vi "DriveZeroRadiusTurnPlanner.vi"(4 "DrivePathPlanParams":T3={"max_velocity (in/s)"=100.0, "max_acceleration (in/s^2)"=80.0, "max_jerk (in/s^3)"=100.0, "dt(ms)"=40, "sample_count"=1000, "wheelbase_width (in)"=25.0} {"dt(ms)" items=["TrajectoryDuration_0ms"=0, "TrajectoryDuration_5ms"=5, "TrajectoryDuration_10ms"=10, "TrajectoryDuration_20ms"=20, "TrajectoryDuration_30ms"=30, "TrajectoryDuration_40ms"=40, "TrajectoryDuration_50ms"=50, "TrajectoryDuration_100ms"=100]}, 5 "Waypoints":T2[](array[typedef])) -> (1 "RightTrajectory":T1[](array[typedef]), 2 "LeftTrajectory":T1[](array[typedef]))   [LabVIEW 2018]
uses:
  PathPlannerSupport/TypeDefs/DrivePathfinderParams.ctl
  <vilib>/Rock Robotics/WPI/ThirdParty/Phoenix-LabVIEW/Motor Controller/Controls/CTRE_Phoenix_MotorControl_TrajectoryPointTimeDur.ctl
  Pathfinder/Pathfinder-LabVIEW/Pathfinder-Lib/VIs/Waypoint.ctl
  Pathfinder/Pathfinder-LabVIEW/Pathfinder-Lib/VIs/Segment.ctl
  General/MotionProfiling/TypeDefs/MotionProfileGeneratorParams.ctl
  Pathfinder/Pathfinder-LabVIEW/Pathfinder-Lib/Pathfinder.lvlib
  ArgosLib/ArgosLib.lvlib
panel:
  in  "Maximum Travel Speed (units/s)":dbl=100.0 format="%#_13g"
  in  "Velocity Ramp Time (ms)":dbl=100.0 format="%#_13g"
  in  "Acceleration Ramp Time (ms)":dbl=200.0 format="%#_13g"
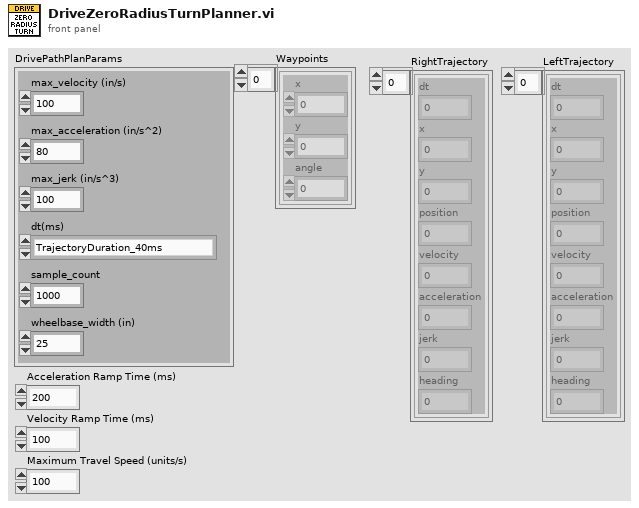
[diagram p1: front panel]
types:
  T1 = typedef "Pathfinder.lvlib/Segment.ctl" = cluster{"dt":dbl, "x":dbl, "y":dbl, "position":dbl, "velocity":dbl, "acceleration":dbl, "jerk":dbl, "heading":dbl}
  T2 = typedef "Pathfinder.lvlib/Waypoint.ctl" = cluster{"x":dbl, "y":dbl, "angle":dbl}
  T3 = typedef "DrivePathfinderParams.ctl" = cluster{"max_velocity (in/s)":dbl, "max_acceleration (in/s^2)":dbl, "max_jerk (in/s^3)":dbl, "dt(ms)":T4, "sample_count":i32, "wheelbase_width (in)":dbl}
  T4 = typedef "CTRE_Phoenix_MotorControl_TrajectoryPointTimeDur.ctl" = i32
  T5 = typedef "MotionProfileGeneratorParams.ctl" = cluster{"Trajectory Point Interval (ms)":T4, "Maximum Travel Speed (units/s)":dbl, "Velocity Ramp Time (ms)":dbl, "Acceleration Ramp Time (ms)":dbl}
  T6 = typedef "TrajectoryPoint.ctl" = cluster{"Position ":dbl, "Velocity ":dbl, "Time (ms)":T4, "Last Point":bool}
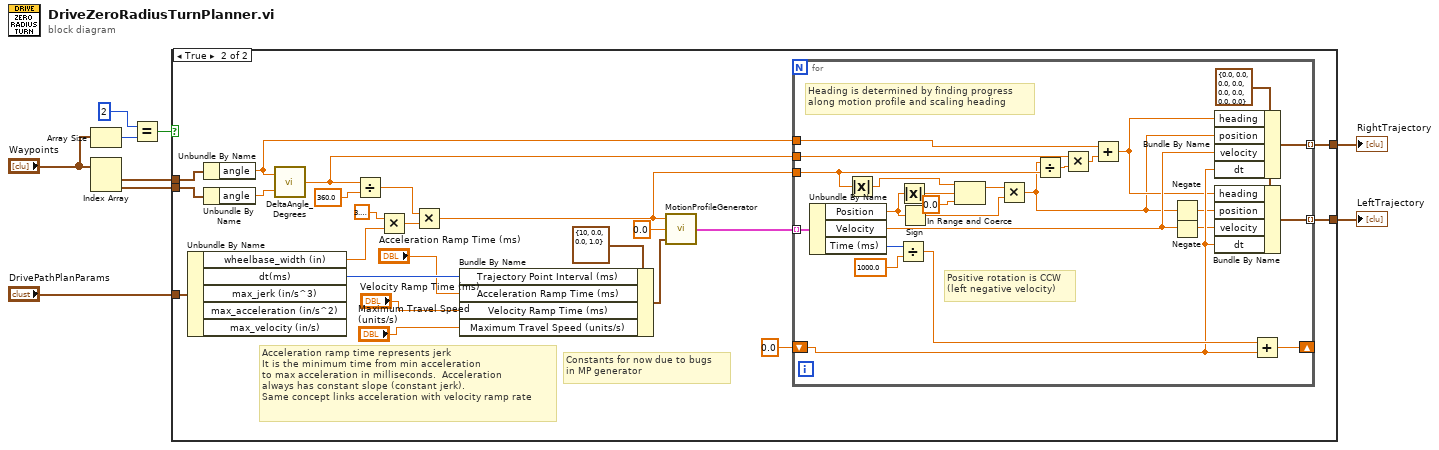
[diagram p0: block diagram]
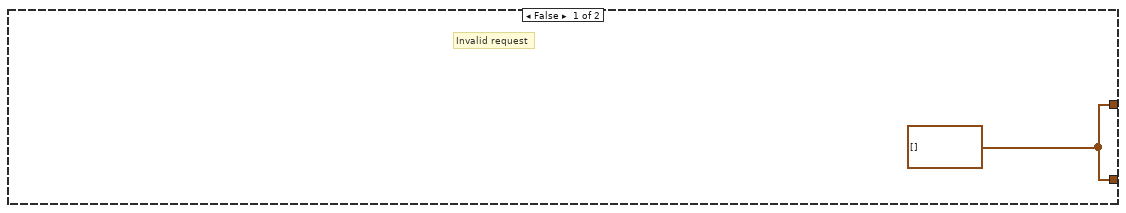
[diagram p2: hidden frame]
diagram:
  n1 = Array Size(array="Waypoints") -> (size(s)=w9:i32)
  n2 = Index Array(array="Waypoints") -> (element #1=w4:T2, element #2=w3:T2)  [unwired: 2 in]
  n3 = Equal?(x=2, y=w9) -> (x = y?=w7:bool)
  n4 = case shown="True" w7 {
    tunnel: [w10 w18] -> w6
    tunnel: w4 -> [_ w32]
    tunnel: w3 -> [_ w31]
    tunnel: "DrivePathPlanParams" -> [_ w33]
    tunnel: [w10 w19] -> w1
    frame False {
      w10 = T1[] [] ("RightTrajectory")
      # "Invalid request"
    }
    frame True {
      # "Constants for now due to bugs\nin MP generator"
      # "Acceleration ramp time represents jerk\nIt is the minimum time from min acceleration\nto max acceleration in milliseconds.  Acceleration\nalways has constant slope (constant jerk).\nSame concept links acceleration with velocity ramp rate"
      n5 = Unbundle By Name(w33) -> ("wheelbase_width (in)"=w23:dbl, "dt(ms)"=w21:T4)  [unwired: 3 out]
      n6 = Unbundle By Name(w32) -> ("angle"=w16:dbl)
      n7 = Unbundle By Name(w31) -> ("angle"=w30:dbl)
      n8 = call "DeltaAngle_Degrees.vi"("EndAngle (deg)"=w30, "StartAngle (deg)"=w16) -> ("DeltaAngle (deg)"=w15:dbl)
      n9 = Divide(x=w15, y=360.0) -> (x/y=w27:dbl)
      n10 = Multiply(x=3.141592653589793, y=w23) -> (x*y=w28:dbl)
      n11 = Multiply(x=w27, y=w28) -> (x*y=w14:dbl)
      n12 = Bundle By Name(cluster=T5 {"Trajectory Point Interval (ms)"=10, "Maximum Travel Speed (units/s)"=0.0, "Velocity Ramp Time (ms)"=0.0, "Acceleration Ramp Time (ms)"=1.0} ("MotionProfileGeneratorParameters"), "Trajectory Point Interval (ms)"=w21, "Acceleration Ramp Time (ms)"="Acceleration Ramp Time (ms)", "Velocity Ramp Time (ms)"="Velocity Ramp Time (ms)", "Maximum Travel Speed (units/s)"="Maximum Travel Speed (units/s)") -> (w24:T5)
      n13 = call "MotionProfileGenerator.vi"("MotionProfileGeneratorParameters"=w24, "Starting Position (units)"=0.0, "Travel Distance (units)"=w14) -> ("Trajectory Points"=w17:T6[])
      n14 = for {
        tunnel: w17 -> [w58] mode=indexing
        shift-right: [w55] -> _
        shift-left: 0.0 -> [w50]
        tunnel: [w53] -> w19 mode=indexing
        tunnel: [w51] -> w18 mode=indexing
        tunnel: w16 -> [w43]
        tunnel: w15 -> [w45]
        tunnel: w14 -> [w38]
        w52 = T1 {"dt"=0.0, "x"=0.0, "y"=0.0, "position"=0.0, "velocity"=0.0, "acceleration"=0.0, "jerk"=0.0, "heading"=0.0} ("segment")
        # "Heading is determined by finding progress\nalong motion profile and scaling heading"
        # "Positive rotation is CCW\n(left negative velocity)"
        n15 = Unbundle By Name(w58) -> ("Position"=w41:dbl, "Velocity"=w48:dbl, "Time (ms)"=w57:T4)
        n16 = Absolute Value(x=w38) -> (abs(x)=w37:dbl)
        n17 = Divide(x=w57, y=1000.0) -> (x/y=w54:dbl)
        n18 = Absolute Value(x=w41) -> (abs(x)=w40:dbl)
        n19 = Sign(1:w41) -> (0:w35:dbl)
        n20 = In Range and Coerce(upper limit=w37, x=w40, lower limit=0.0) -> (coerced(x)=w36:dbl)  [unwired: 1 out]
        n21 = Multiply(x=w36, y=w35) -> (x*y=w34:dbl)
        n22 = Divide(x=w34, y=w38) -> (x/y=w46:dbl)
        n23 = Multiply(x=w45, y=w46) -> (x*y=w44:dbl)
        n24 = Add(x=w43, y=w44) -> (x+y=w42:dbl)
        n25 = Negate(x=w34) -> (-x=w49:dbl)
        n26 = Negate(x=w48) -> (-x=w47:dbl)
        n27 = Bundle By Name(cluster=w52, "heading"=w42, "position"=w34, "velocity"=w48, "dt"=w50) -> (w53:T1)
        n28 = Bundle By Name(cluster=w52, "heading"=w42, "position"=w49, "velocity"=w47, "dt"=w50) -> (w51:T1)
        n29 = Add(x=w54, y=w50) -> (x+y=w55:dbl)
      }
    }
  }
  "RightTrajectory" <- w1
  "LeftTrajectory" <- w6
